vi "fgv_joystick_remote.vi"(7 "cmd":enum16{"ini", "read", "close"}(ring), 8 "error in":errorcluster) -> (0 "error out":errorcluster, 3 "joystick info-out":T1)   [LabVIEW 2019]
uses:
  Ctrl/cmd_common.ctl
  <vilib>/Utility/inputDevices.llb/joystickAcquire.vi
  <vilib>/Utility/inputDevices.llb/closeJoystick.vi
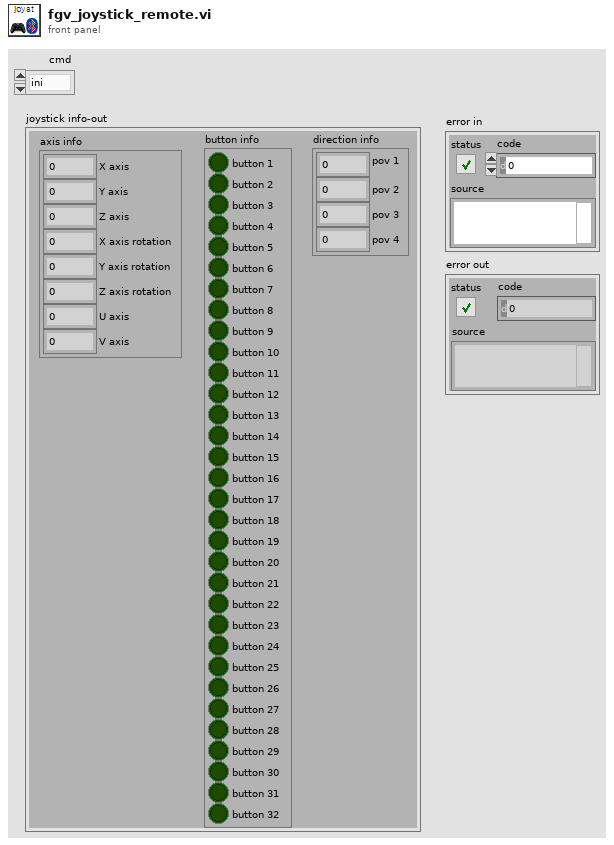
[diagram p1: front panel]
types:
  T1 = cluster{"axis info":cluster{"X axis":i32, "Y axis":i32, "Z axis":i32, "X axis rotation":i32, "Y axis rotation":i32, "Z axis rotation":i32, "U axis":i32, "V axis":i32}, "button info":cluster{"button 1":bool, "button 2":bool, "button 3":bool, "button 4":bool, "button 5":bool, "button 6":bool, "button 7":bool, "button 8":bool, "button 9":bool, "button 10":bool, "button 11":bool, "button 12":bool, "button 13":bool, "button 14":bool, "button 15":bool, "button 16":bool, "button 17":bool, "button 18":bool, "button 19":bool, "button 20":bool, "button 21":bool, "button 22":bool, "button 23":bool, "button 24":bool, "button 25":bool, "button 26":bool, "button 27":bool, "button 28":bool, "button 29":bool, "button 30":bool, "button 31":bool, "button 32":bool}, "direction info":cluster{"pov 1":i32, "pov 2":i32, "pov 3":i32, "pov 4":i32}}
  T2 = typedef "cmd_common.ctl" = enum16{"read", "write"}
  T3 = typedef "joystick cfg.ctl" = cluster{"Type":enum16{"Logitech F710", "Xbox"}, "steer limit":cluster{"min":dbl, "max":dbl, "scale":dbl, "offset":dbl}, "speed limit":cluster{"min":dbl, "max":dbl, "pwm max":dbl}, "ID":i32, "joystick max":dbl}
  T4 = cluster{"X axis":i32, "Y axis":i32, "Z axis":i32, "X axis rotation":i32, "Y axis rotation":i32, "Z axis rotation":i32, "U axis":i32, "V axis":i32}
  T5 = cluster{"button 1":bool, "button 2":bool, "button 3":bool, "button 4":bool, "button 5":bool, "button 6":bool, "button 7":bool, "button 8":bool, "button 9":bool, "button 10":bool, "button 11":bool, "button 12":bool, "button 13":bool, "button 14":bool, "button 15":bool, "button 16":bool, "button 17":bool, "button 18":bool, "button 19":bool, "button 20":bool, "button 21":bool, "button 22":bool, "button 23":bool, "button 24":bool, "button 25":bool, "button 26":bool, "button 27":bool, "button 28":bool, "button 29":bool, "button 30":bool, "button 31":bool, "button 32":bool}
  T6 = cluster{"pov 1":i32, "pov 2":i32, "pov 3":i32, "pov 4":i32}
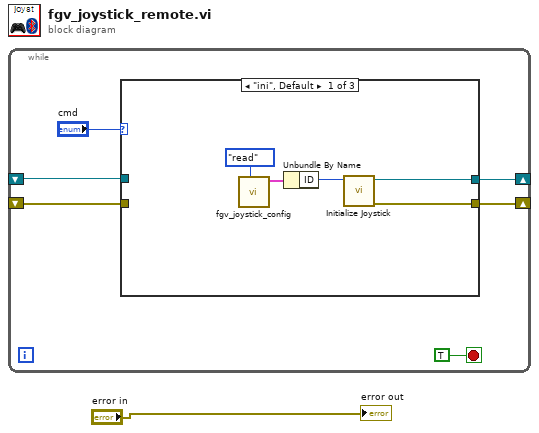
[diagram p0: block diagram]
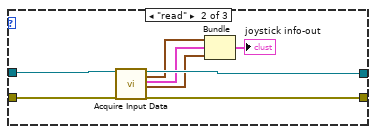
[diagram p2: hidden frame]
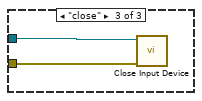
[diagram p3: hidden frame]
diagram:
  n1 = while {
    shift-right: [w5] -> _
    shift-left: _ -> [w3]
    shift-right: [w4] -> _
    shift-left: _ -> [w2]
    stop <- TRUE stop-if-true
    n2 = case shown="\"ini\", Default" "cmd" {
      tunnel: [w12 w20 _] -> w5
      tunnel: [w11 w19 _] -> w4
      tunnel: w3 -> [_ w18 w22]
      tunnel: w2 -> [_ w17 w21]
      frame "ini", Default {
        n3 = call "fgv_joystick_config.vi"("cmd"=cmd_common."read") -> ("Joystick cfg out"=w9:T3)  [unwired: 9 in, 1 out]
        n4 = Unbundle By Name(w9) -> ("ID"=w8:i32)
        n5 = call <vilib>:"Initialize Joystick.vi"("device index"=w8) -> ("error out"=w11:errorcluster, "device ID"=w12:refnum<k1>)  [unwired: 9 in]
      }
      frame "read" {
        n6 = call-poly <vilib>:"Acquire Input Data.vi"("device ID"=w18, "error in (no error)"=w17) -> ("device ID"=w20:refnum<k1>, "axis info"=w14:T4, "button info"=w15:T5, "direction info"=w16:T6, "error out"=w19:errorcluster)  [unwired: 13 in]
        n7 = Bundle("axis info"=w14, "button info"=w15, "direction info"=w16) -> (→"joystick info-out":T1)  [unwired: 1 in]
      }
      frame "close" {
        n8 = call-poly <vilib>:"Close Input Device.vi"("error in (no error)"=w21, "device ID"=w22) -> ()  [unwired: 8 in, 1 out]
      }
    }
  }
  "error out" <- "error in"
